vi "SQLite3 Error Cluster From Error Code.vi"(4 "is warning? (False)":bool, 5 "show call chain? (False)":bool, 6 "error in (no error)":errorcluster, 8 "error message (\"\")":string, 9 "error code (0)":i32) -> (0 "error out":errorcluster)   [LabVIEW 2014, in "SQLite3LV.lvlib"]
doc: "Converts an error or warning code to an error cluster. This VI is useful when you receive a return value from a shared library call or when you return user-defined error codes."
uses:
  SQLite3LV.lvlib
  <vilib>/Utility/error.llb/whitespace.ctl
panel:
  in  "call chain header":string="\n<b>Complete call chain:</b>"
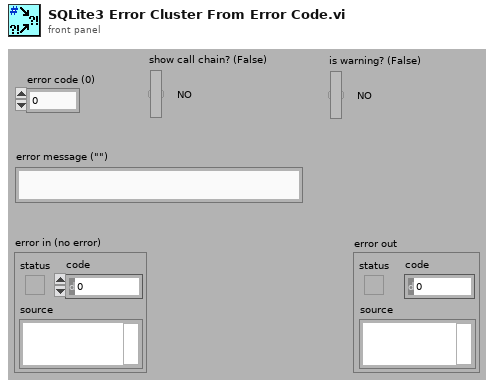
[diagram p1: front panel]
types:
  T1 = typedef "whitespace.ctl" = u16
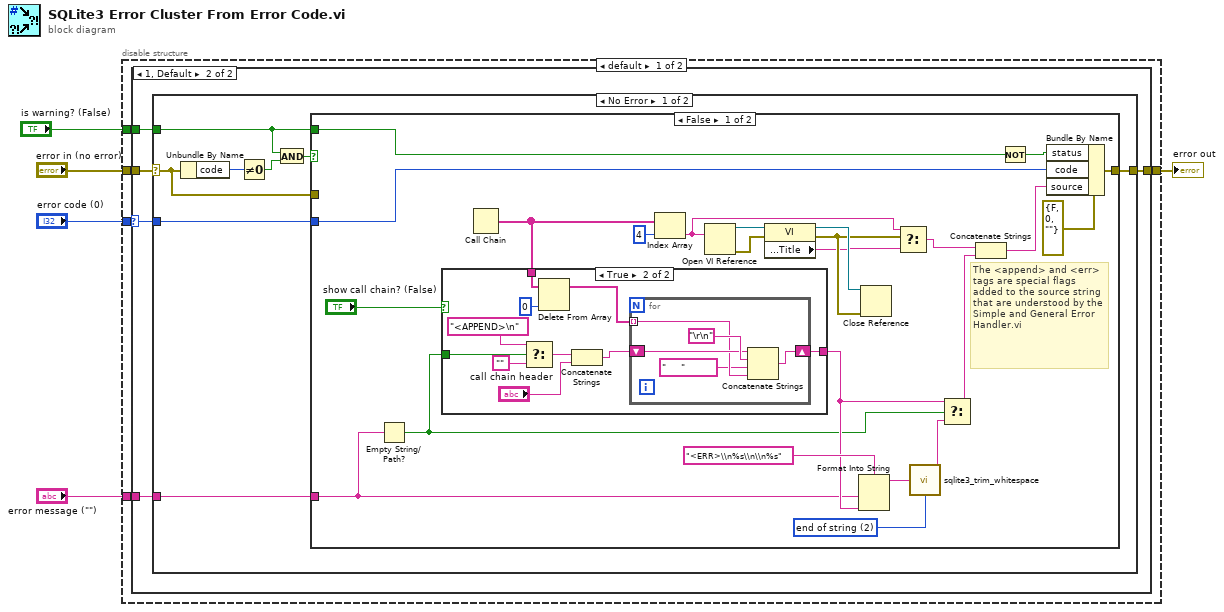
[diagram p0: block diagram]
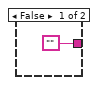
[diagram p3: hidden frame]
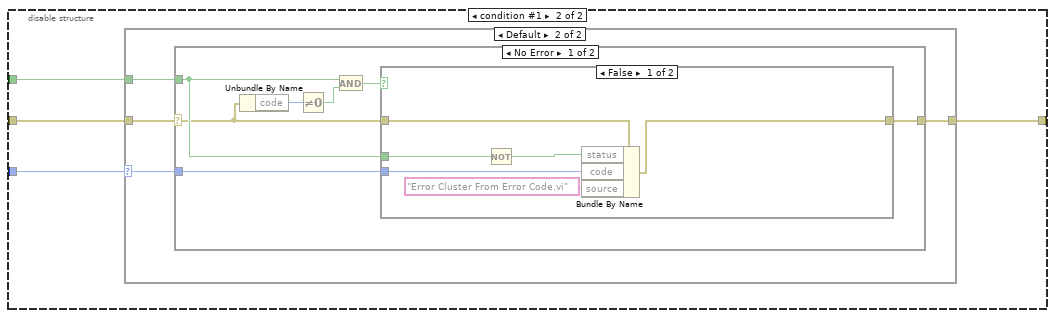
[diagram p6: hidden frame]
diagram:
  n1 = disable-structure shown="default" {
    disable-tunnel: [w10 w69] -> w5
    disable-tunnel: "error in (no error)" -> [w9 w70]
    disable-tunnel: "error code (0)" -> [w8 w68]
    disable-tunnel: "error message (\"\")" -> [w7 _]
    disable-tunnel: "is warning? (False)" -> [w6 w67]
    frame condition #0 (active) {
      n2 = case shown="1, Default" w8 {
        selector: w8 -> [_ w14]
        tunnel: [w11 w16] -> w10
        tunnel: w9 -> [w11 w15]
        tunnel: w7 -> [_ w13]
        tunnel: w6 -> [_ w12]
        frame 0 {
          # "If the error code in equals zero, then propagate the error in cluster regardless of its value."
        }
        frame 1, Default {
          n3 = case shown="No Error" w15 {
            selector: w15 -> [w19 w66]
            tunnel: [w24 w66] -> w16
            tunnel: w14 -> [w23 _]
            tunnel: w13 -> [w18 _]
            tunnel: w12 -> [w17 _]
            frame No Error {
              n4 = Unbundle By Name(w19) -> ("code"=w22:i32)
              n5 = Not Equal To 0?(x=w22) -> (x != 0?=w20:bool)
              n6 = And(x=w17, y=w20) -> (x .and. y?=w21:bool)
              n7 = case shown="False" w21 {
                tunnel: [w48 w65] -> w24
                tunnel: w23 -> [w44 _]
                tunnel: w19 -> [_ w65]
                tunnel: w17 -> [w34 _]
                tunnel: w18 -> [w29 _]
                frame False {
                  w25 = T1 2 items=["both", "start of string", "end of string"] ("location (both)")
                  # "The <append> and <err> tags are special flags added to the source string that are understood by the Simple and General Error Handler.vi"
                  n8 = Empty String/Path?(string/path=w29) -> (empty?=w28:bool)
                  n9 = Call Chain() -> (call chain=w39:string[])
                  n10 = case shown="True" "show call chain? (False)" {
                    tunnel: ["" w59] -> w31
                    tunnel: w39 -> [_ w57]
                    tunnel: w28 -> [_ w53]
                    frame False {
                    }
                    frame True {
                      n11 = Select(t="<APPEND>\n", s=w53, f="") -> (s? t:f=w50:string)
                      n12 = Delete From Array(array=w57, index=0) -> (array with subset deleted=w56:string[])  [unwired: 1 in, 1 out]
                      n13 = Concatenate Strings(w50, "call chain header") -> (w54:string)
                      n14 = for {
                        tunnel: w56 -> [w61] mode=indexing
                        shift-right: [w64] -> w59
                        shift-left: w54 -> [w62]
                        n15 = Concatenate Strings(w62, "\r\n", "     ", w61) -> (w64:string)
                      }
                    }
                  }
                  n16 = Index Array(array=w39, index=4) -> (element=w37:string)
                  n17 = Open VI Reference(vi path=w37) -> (vi reference=w42:refnum<vi>, error out=w41:errorcluster)  [unwired: 5 in]
                  n18 = property class="VI"(reference=w42, error in=w41) -> (reference out=w40:refnum<vi>, error out=w38:errorcluster, "Front Panel Window:Title"=w36:string)
                  n19 = Format Into String(format string="<ERR>\\n%s\\n\\n%s", w29, w31) -> (resulting string=w27:string)  [unwired: 2 in, 1 out]
                  n20 = Close Reference(reference=w40, error in (no error)=w38) -> ()  [unwired: 1 out]
                  n21 = Select(t=w37, s=w38, f=w36) -> (s? t:f=w35:string)
                  n22 = call "sqlite3_trim_whitespace.vi"("string"=w27, "location (both)"=w25) -> ("trimmed string"=w26:string)
                  n23 = Select(t=w31, s=w28, f=w26) -> (s? t:f=w30:string)
                  n24 = Concatenate Strings(w35, w30) -> (w46:string)
                  n25 = Not(x=w34) -> (.not. x?=w45:bool)
                  n26 = Bundle By Name(cluster=errorcluster {"status"=FALSE, "code"=0, "source"=""} ("error out"), "status"=w45, "code"=w44, "source"=w46) -> (w48:errorcluster)
                }
                frame True {
                  # "If the error code input is setting a warning, and a warning is already set on the wire, then we\ngo with the one already on the wire."
                }
              }
            }
            frame Error {
              # "An error in trumps any error code input."
            }
          }
        }
      }
    }
    frame condition #1 {
      n27 = case shown="Default" w68 {
        selector: w68 -> [_ w73]
        tunnel: w70 -> [w71 w75]
        tunnel: [w71 w74] -> w69
        tunnel: w67 -> [_ w72]
        frame 0 {
          # "If the error code in equals zero, then propagate the error in cluster regardless of its value."
        }
        frame Default {
          n28 = case shown="No Error" w75 {
            selector: w75 -> [w77 w90]
            tunnel: [w81 w90] -> w74
            tunnel: w73 -> [w82 _]
            tunnel: w72 -> [w78 _]
            frame No Error {
              n29 = Unbundle By Name(w77) -> ("code"=w80:i32)
              n30 = Not Equal To 0?(x=w80) -> (x != 0?=w79:bool)
              n31 = And(x=w78, y=w79) -> (x .and. y?=w76:bool)
              n32 = case shown="False" w76 {
                tunnel: w82 -> [w88 _]
                tunnel: [w85 w89] -> w81
                tunnel: w78 -> [w84 _]
                tunnel: w77 -> [w83 w89]
                frame False {
                  n33 = Not(x=w84) -> (.not. x?=w87:bool)
                  n34 = Bundle By Name(cluster=w83, "status"=w87, "code"=w88, "source"="Error Cluster From Error Code.vi") -> (w85:errorcluster)
                }
                frame True {
                  # "If the error code input is setting a warning, and a warning is already set on the wire, then we\ngo with the one already on the wire."
                }
              }
            }
            frame Error {
              # "An error in trumps any error code input."
            }
          }
        }
      }
    }
  }
  "error out" <- w5
